vi "Update Children.vi"(6 "Labels":map{string, string}(c390), 8 "error in (no error)":errorcluster, 9 "Created?":bool=TRUE, 10 "New Value":dbl, 11 "Histogram in":refnum<class "Histogram.lvclass">) -> (0 "error out":errorcluster, 3 "Histogram out":refnum<class "Histogram.lvclass">)   [LabVIEW 2020, in "Metrics.lvlib" / "Histogram.lvclass"]
uses:
  Histogram.lvclass
  Histogram.lvclass/Histogram.ctl
  metric/Metric.lvclass/Metric.ctl
  <vilib>/Utility/miscctls.llb/LVMapReplaceAction.ctl
  sample/Edit Action.ctl
  metric/Read Samples.vi
  metric/Write Samples 2.vi
  sample/Sample.lvclass
  metric/Metric.lvclass
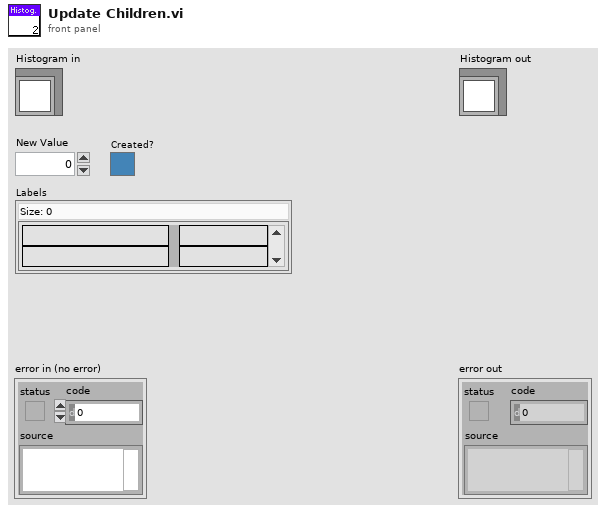
[diagram p1: front panel]
types:
  T1 = typedef "LVMapReplaceAction.ctl" = enum32{"Modify Entry only if found", "Add or Modify Entry", "Delete Entry"}
  T2 = typedef "Metrics.lvlib/Sample.lvclass/Edit Action.ctl" = enum16{"Set", "Increment"}
  T3 = enum16{"seconds", "milliseconds", "microseconds"}
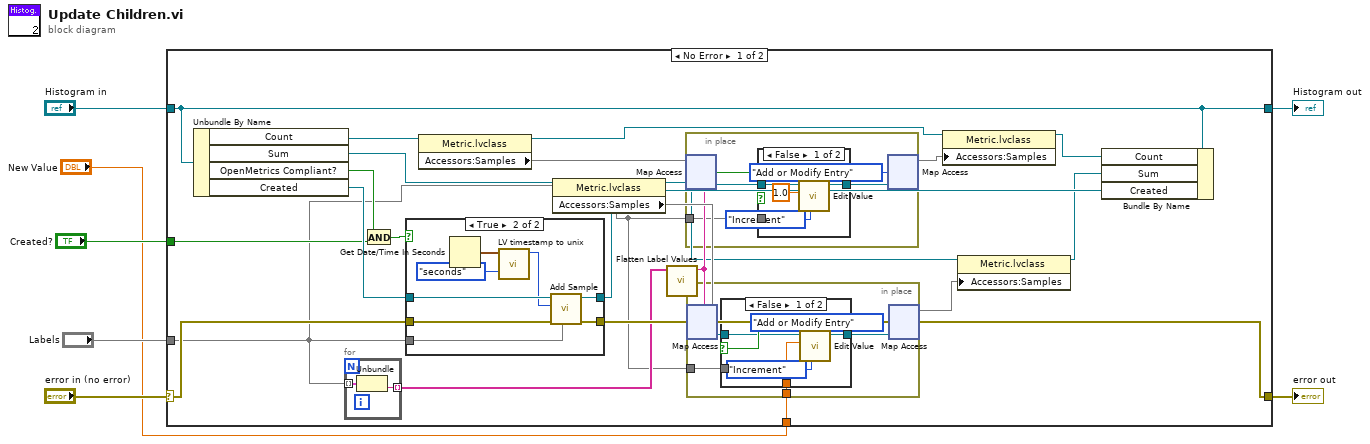
[diagram p0: block diagram]
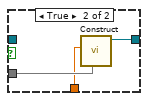
[diagram p2: hidden frame]
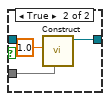
[diagram p3: hidden frame]
diagram:
  n1 = case shown="No Error" "error in (no error)" {
    selector: "error in (no error)" -> [w26 w68]
    tunnel: [w25 w68] -> w6
    tunnel: [w27 w67] -> w4
    tunnel: "Histogram in" -> [w27 w67]
    tunnel: "Labels" -> [w9 _]
    tunnel: "Created?" -> [w24 _]
    tunnel: "New Value" -> [w8 _]
    frame No Error {
      n2 = Unbundle By Name(w27) -> ("Count"=w20:refnum<class "Metric.lvclass">, "Sum"=w18:refnum<class "Metric.lvclass">, "OpenMetrics Compliant?"=w23:bool, "Created"=w28:refnum<class "Metric.lvclass">)
      n3 = for {
        tunnel: w9 -> [w56] mode=indexing
        tunnel: [w55] -> w21 mode=indexing
        n4 = Unbundle(w56) -> (w55:string)  [unwired: 1 out]
      }
      n5 = And(x=w23, y=w24) -> (x .and. y?=w22:bool)
      n6 = case shown="True" w22 {
        tunnel: w28 -> [w58 w66]
        tunnel: w9 -> [_ w62]
        tunnel: [w58 w61] -> w29
        tunnel: w26 -> [w57 w59]
        tunnel: [w57 w60] -> w25
        frame False {
        }
        frame True {
          n7 = Get Date/Time In Seconds() -> (seconds since 1Jan1904=w65:timestamp)
          n8 = call "LV timestamp to unix.vi"("Precision (ms)"=T3."seconds", "Timestamp"=w65) -> ("Unix epoch time"=w63:u64)  [unwired: 9 in]
          n9 = call-dynamic "Add Sample.vi"("Labels"=w62, "error in (no error)"=w59, "Value"=w63, "Metric in"=w66) -> ("error out"=w60:errorcluster, "Metric out"=w61:refnum<class "Metric.lvclass">)  [unwired: 6 in]
        }
      }
      n10 = property class="Metric.lvclass"(reference=w20) -> (reference out=w15:refnum<class "Metric.lvclass">, "Accessors:Samples"=w19:map{string, refnum<class "Sample.lvclass">})  [unwired: 1 in, 1 out]
      n11 = property class="Metric.lvclass"(reference=w18) -> (reference out=w11:refnum<class "Metric.lvclass">, "Accessors:Samples"=w17:map{string, refnum<class "Sample.lvclass">})  [unwired: 1 in, 1 out]
      n12 = call "Flatten Label Values.vi"("Label Values"=w21) -> ("Flattened labelvalues"=w16:string)  [unwired: 10 in]
      n13 = in-place {
        in-place-border: w9 -> [w44]
        n14 = in-place-map #1(w19, w16) -> (w47:refnum<class "Sample.lvclass">, w46:bool)  [unwired: 1 in]
        n15 = case shown="False" w46 {
          tunnel: w47 -> [w51 _]
          tunnel: [w50 w54] -> w45
          tunnel: w44 -> [_ w52]
          frame False {
            n16 = call "Edit Value.vi"("Action"=Edit_Action."Increment", "New Val"=1.0, "Sample in"=w51) -> ("Sample out"=w50:refnum<class "Sample.lvclass">)  [unwired: 7 in, 1 out]
          }
          frame True {
            n17 = call "Construct.vi"("Labels"=w52, "Value"=1.0) -> ("Sample out"=w54:refnum<class "Sample.lvclass">)  [unwired: 8 in, 1 out]
          }
        }
        n18 = in-place-map #1(w45, LVMapReplaceAction."Add or Modify Entry" ("action")) -> (w14:map{string, refnum<class "Sample.lvclass">})  [unwired: 2 out]
      }
      n19 = in-place {
        in-place-border: w9 -> [w32]
        in-place-border: w8 -> [w31]
        n20 = in-place-map #2(w17, w16) -> (w35:refnum<class "Sample.lvclass">, w34:bool)  [unwired: 1 in]
        n21 = case shown="False" w34 {
          tunnel: w35 -> [w39 _]
          tunnel: [w38 w42] -> w33
          tunnel: w32 -> [_ w41]
          tunnel: w31 -> [w37 w40]
          frame False {
            n22 = call "Edit Value.vi"("Action"=Edit_Action."Increment", "New Val"=w37, "Sample in"=w39) -> ("Sample out"=w38:refnum<class "Sample.lvclass">)  [unwired: 7 in, 1 out]
          }
          frame True {
            n23 = call "Construct.vi"("Labels"=w41, "Value"=w40) -> ("Sample out"=w42:refnum<class "Sample.lvclass">)  [unwired: 8 in, 1 out]
          }
        }
        n24 = in-place-map #2(w33, LVMapReplaceAction."Add or Modify Entry" ("action")) -> (w12:map{string, refnum<class "Sample.lvclass">})  [unwired: 2 out]
      }
      n25 = property class="Metric.lvclass"(reference=w15, "Accessors:Samples"=w14) -> (reference out=w13:refnum<class "Metric.lvclass">)  [unwired: 1 in, 1 out]
      n26 = property class="Metric.lvclass"(reference=w11, "Accessors:Samples"=w12) -> (reference out=w10:refnum<class "Metric.lvclass">)  [unwired: 1 in, 1 out]
      n27 = Bundle By Name(cluster=w27, "Count"=w13, "Sum"=w10, "Created"=w29) -> ()  [unwired: 1 out]
    }
    frame Error {
    }
  }
  "error out" <- w6
  "Histogram out" <- w4
